vi "6-2 Read.vi"() -> ()   [LabVIEW 2017]
uses:
  Global 1.vi
panel:
  out "Waveform Chart":dbl(graph)
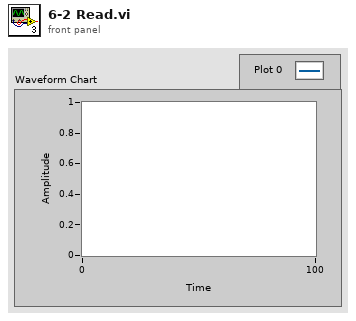
[diagram p1: front panel]
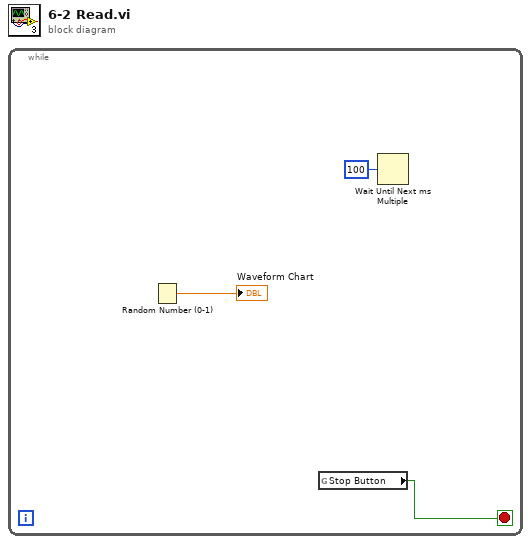
[diagram p0: block diagram]
diagram:
  n1 = while {
    stop <- w3 stop-if-true
    n2 = Random Number (0-1)() -> (number: 0 to 1=→"Waveform Chart":dbl)
    n3 = global read "Global 1.vi" "Stop Button"() -> (w3:bool)
    n4 = Wait Until Next ms Multiple(millisecond multiple=u32 100) -> ()  [unwired: 1 out]
  }
